vi "Known Tags.vi"(7 "Tag Cmd":T1, 8 "error in (no error)":errorcluster, 9 "ini Path":path=path "E:/Mark's Data/OneDrive/Documents/LabVIEW Projects/ComicCleaner/Main.vi", 11 "New Tag":string) -> (0 "error out":errorcluster, 3 "Tag Set":set{string}(c389))   [LabVIEW 2023]
uses:
  TypeDefs/Tag Cmd.ctl
  <vilib>/Utility/config.llb/Write Key (Boolean).vi
  <vilib>/Utility/config.llb/NI_LVConfig.lvlib
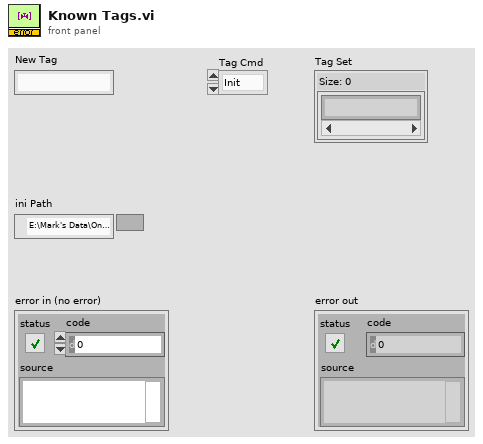
[diagram p1: front panel]
types:
  T1 = typedef "Tag Cmd.ctl" = enum16{"Init", "Get Known", "Set Known"}
  T2 = typedef "NI_LVConfig.lvlib/Config Data RefNum.ctl" = refnum<k1>
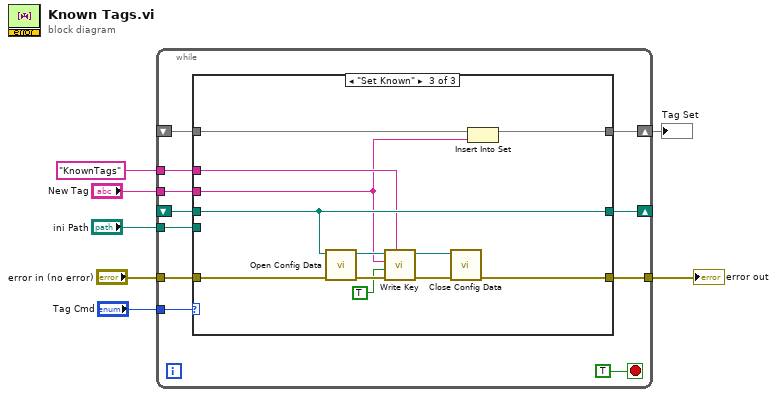
[diagram p0: block diagram]
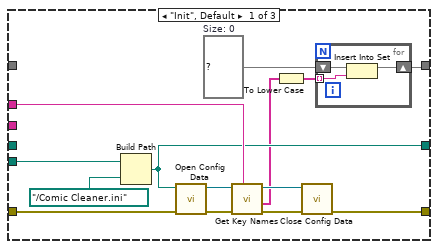
[diagram p2: hidden frame]
diagram:
  n1 = while {
    tunnel: "Tag Cmd" -> [w18]
    tunnel: "error in (no error)" -> [w16]
    tunnel: "ini Path" -> [w15]
    tunnel: "KnownTags" ("section") -> [w14]
    tunnel: [w13] -> w3
    shift-right: [w12] -> _
    shift-left: _ -> [w11]
    tunnel: "New Tag" -> [w10]
    shift-right: [w9] -> w1
    shift-left: _ -> [w8]
    stop <- TRUE stop-if-true
    n2 = case shown="\"Set Known\"" w18 {
      tunnel: w16 -> [w32 w37 w50]
      tunnel: w15 -> [w31 _ _]
      tunnel: w14 -> [w28 _ w42]
      tunnel: [w25 w37 w43] -> w13
      tunnel: [w24 w38 w49] -> w12
      tunnel: w11 -> [_ w38 w49]
      tunnel: w10 -> [_ _ w39]
      tunnel: [w22 w36 w41] -> w9
      tunnel: w8 -> [_ w36 w40]
      frame "Init", Default {
        w20 = set{string} {}  # Size: 0
        n3 = Build Path(base path=w31, name or relative path=path "../Comic Cleaner.ini") -> (appended path=w24:path)
        n4 = call <vilib>:"Open Config Data.vi"("error in (no error)"=w32, "configuration file path"=w24) -> ("error out"=w30:errorcluster, "refnum"=w29:T2)  [unwired: 7 in, 1 out]
        n5 = call <vilib>:"Get Key Names.vi"("section"=w28, "error in (no error)"=w30, "refnum"=w29) -> ("error out"=w26:errorcluster, "key names"=w21:string[], "refnum out"=w27:T2)  [unwired: 5 in, 1 out]
        n6 = To Lower Case(string=w21) -> (all lower case string=w19:string[])
        n7 = call <vilib>:"Close Config Data.vi"("error in (no error)"=w26, "refnum"=w27) -> ("error out"=w25:errorcluster)  [unwired: 8 in, 1 out]
        n8 = for {
          shift-right: [w35] -> w22
          shift-left: w20 -> [w34]
          tunnel: w19 -> [w33] mode=indexing
          n9 = Insert Into Set(10:w33, 11:w34) -> (3:w35:set{string})  [unwired: 1 out]
        }
      }
      frame "Get Known" {
      }
      frame "Set Known" {
        n10 = call <vilib>:"Open Config Data.vi"("error in (no error)"=w50, "configuration file path"=w49) -> ("error out"=w48:errorcluster, "refnum"=w47:T2)  [unwired: 7 in, 1 out]
        n11 = call-poly <vilib>:"Write Key.vi"("section"=w42, "error in (no error)"=w48, "value"=TRUE, "key"=w39, "refnum"=w47) -> ("error out"=w45:errorcluster, "refnum out"=w44:T2)  [unwired: 4 in, 1 out]
        n12 = call <vilib>:"Close Config Data.vi"("error in (no error)"=w45, "refnum"=w44) -> ("error out"=w43:errorcluster)  [unwired: 8 in, 1 out]
        n13 = Insert Into Set(10:w39, 11:w40) -> (3:w41:set{string})  [unwired: 1 out]
      }
    }
  }
  "error out" <- w3
  "Tag Set" <- w1
